vi "LPF (SubVI).vi"(9 "ZeroDimension":i32=4000, 10 "ФНЧ":bool, 11 "In":dbl[](array[numeric])) -> (3 "Filtered X":dbl[](array[numeric]))   [LabVIEW 2017]
uses:
  <vilib>/Analysis/NI_AALPro.lvlib
  <vilib>/Analysis/NI_AALBase.lvlib
panel:
  in  "Echo":bool
  in  "first":i32
  in  "Position":i32=2050
  in  "amplitude":dbl=0.002 format="%.2p"
  in  "cycles":dbl=2.0 format="%#_13g"
  in  "samples":i32=20
  in  "last":i32
  in  "index":i32
  out "Waveform Graph":dbl[][](graph)
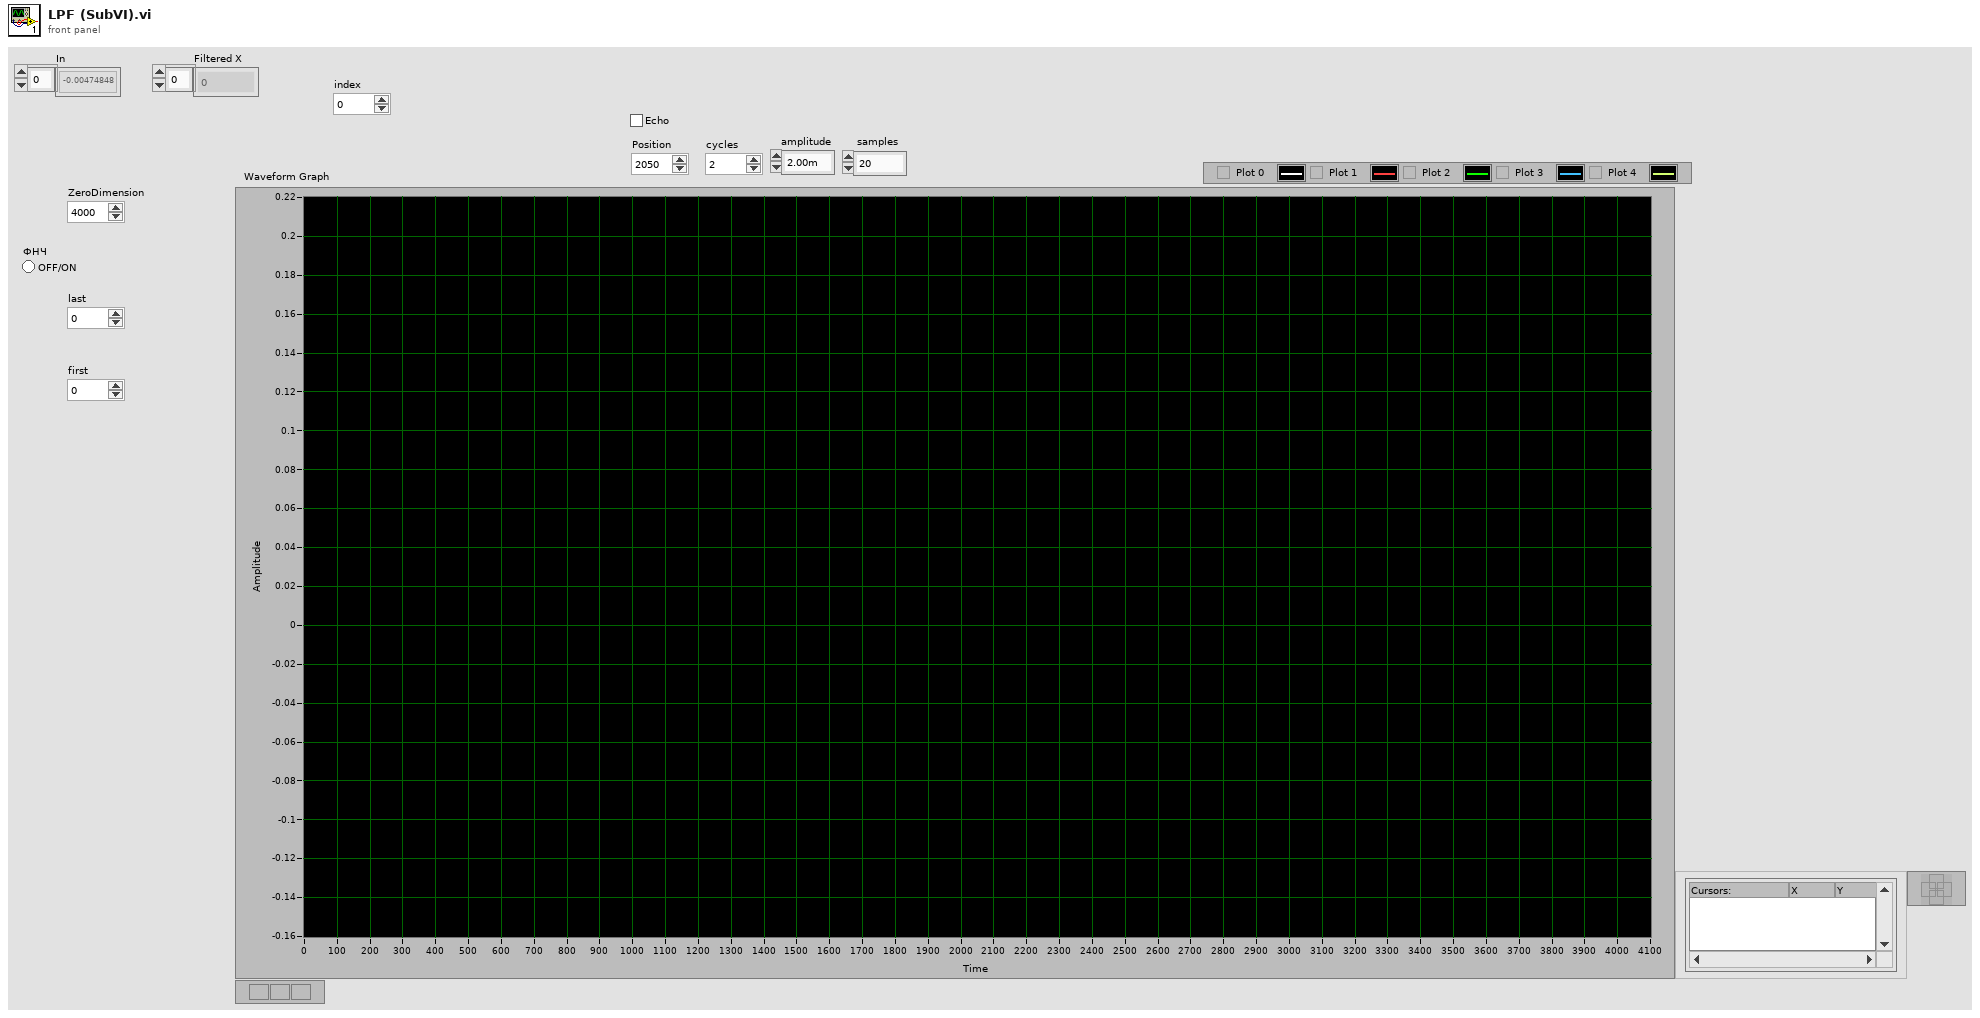
[diagram p1: front panel]
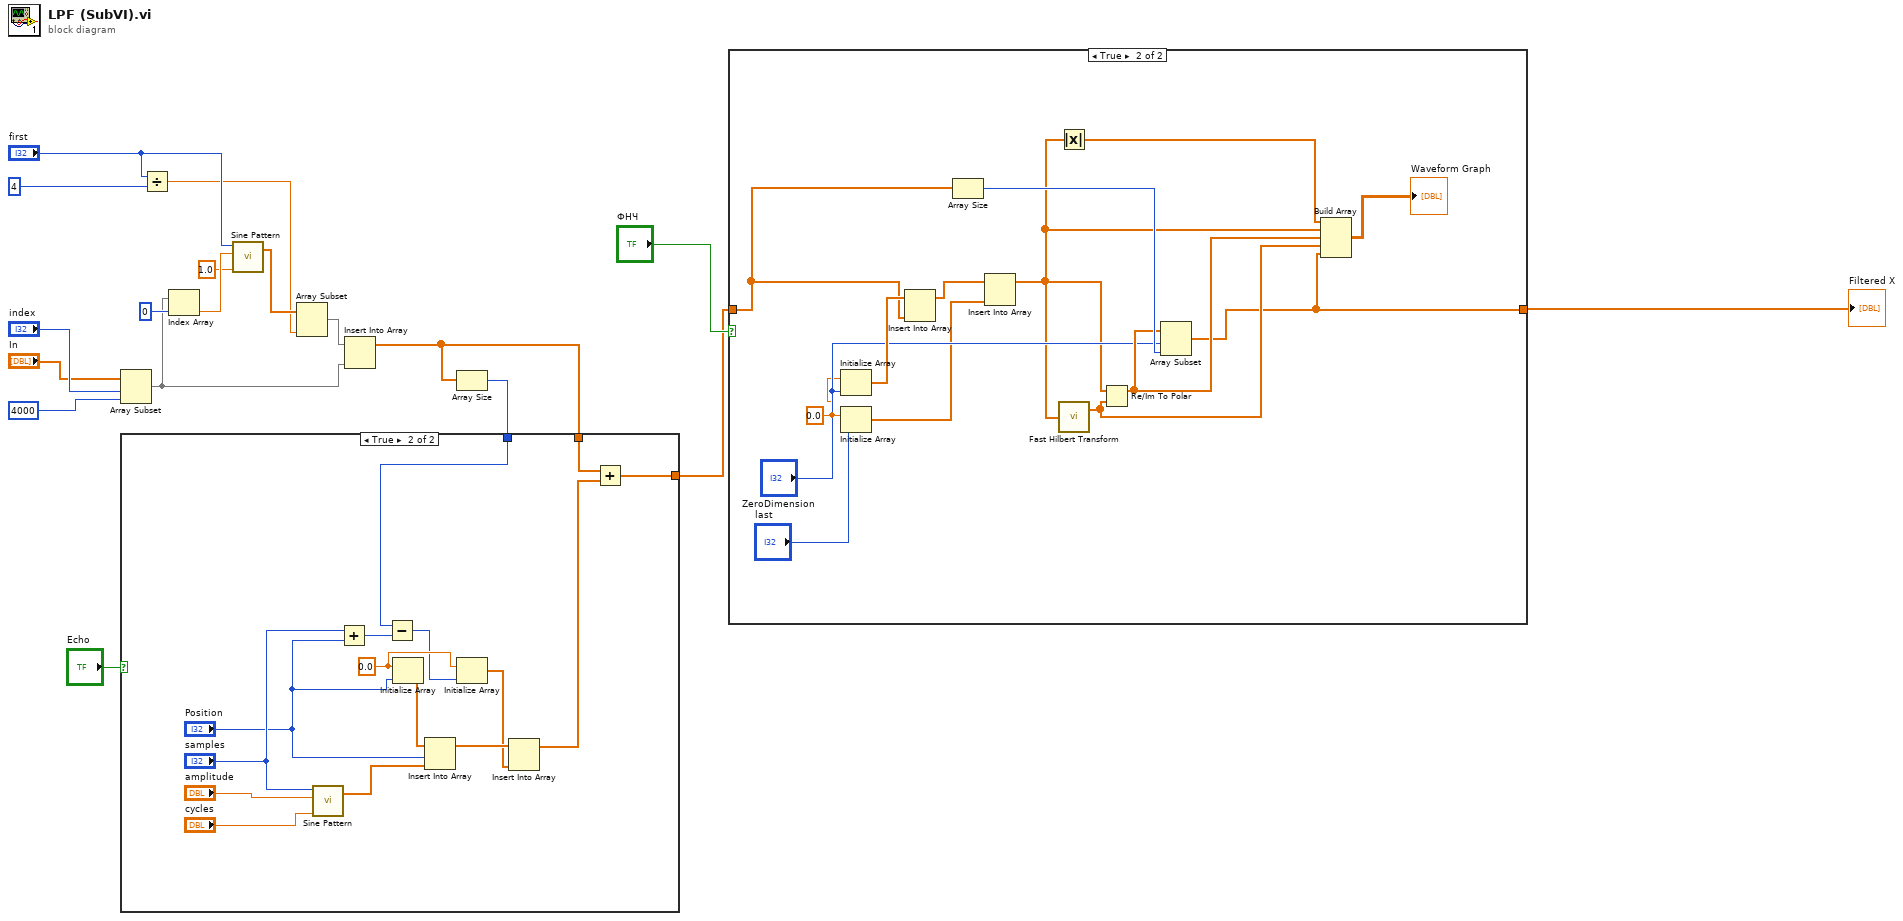
[diagram p0: block diagram]
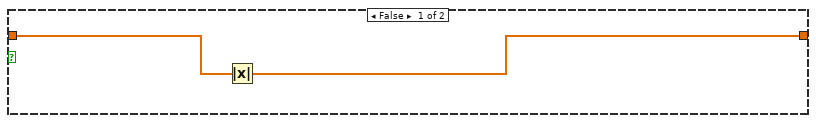
[diagram p3: hidden frame]
diagram:
  n1 = Array Subset(array="In", index="index", length=4000) -> (w3:dbl[])
  n2 = Divide(x="first", y=4) -> (x/y=w5:dbl)
  n3 = Index Array(array=w3, index=0) -> (element=w10:dbl)
  n4 = call <vilib>:"Sine Pattern.vi"("cycles"=1.0, "amplitude"=w10, "samples"="first") -> ("Sinusoidal Pattern"=w8:dbl[])  [unwired: 1 in, 1 out]
  n5 = Array Subset(array=w8, length=w5) -> (w4:dbl[])  [unwired: 1 in]
  n6 = Insert Into Array(array=w4, new element=w3) -> (w2:dbl[])  [unwired: 1 in]
  n7 = Array Size(array=w2) -> (size(s)=w13:i32)
  n8 = case shown="True" "Echo" {
    tunnel: w13 -> [_ w29]
    tunnel: [w19 w21] -> w12
    tunnel: w2 -> [w19 w20]
    frame False {
    }
    frame True {
      w30 = 0.0 ("element")
      n9 = call <vilib>:"Sine Pattern.vi"("cycles"="cycles", "amplitude"="amplitude", "samples"="samples") -> ("Sinusoidal Pattern"=w32:dbl[])  [unwired: 1 in, 1 out]
      n10 = Add(x="samples", y="Position") -> (x+y=w26:i32)
      n11 = Subtract(x=w29, y=w26) -> (x-y=w25:i32)
      n12 = Initialize Array(w30, "Position") -> (w31:dbl[])
      n13 = Insert Into Array(array=w31, index="Position", new element=w32) -> (w24:dbl[])
      n14 = Initialize Array(w30, w25) -> (w23:dbl[])
      n15 = Insert Into Array(array=w24, new element=w23) -> (w22:dbl[])  [unwired: 1 in]
      n16 = Add(x=w20, y=w22) -> (x+y=w21:dbl[])
    }
  }
  n17 = case shown="True" "ФНЧ" {
    tunnel: w12 -> [w36 w46]
    tunnel: [w35 w37] -> w17
    frame False {
      n18 = Absolute Value(x=w36) -> (abs(x)=w35:dbl[])
    }
    frame True {
      w40 = 0.0 ("element")
      n19 = Initialize Array(w40, "ZeroDimension") -> (w49:dbl[])
      n20 = Initialize Array(w40, "last") -> (w44:dbl[])
      n21 = Insert Into Array(array=w49, new element=w46) -> (w48:dbl[])  [unwired: 1 in]
      n22 = Array Size(array=w46) -> (size(s)=w50:i32)
      n23 = Insert Into Array(array=w48, new element=w44) -> (w39:dbl[])  [unwired: 1 in]
      n24 = Absolute Value(x=w39) -> (abs(x)=w38:dbl[])
      n25 = call <vilib>:"Fast Hilbert Transform.vi"("X"=w39) -> ("Hilbert{X}"=w42:dbl[])  [unwired: 1 out]
      n26 = Re/Im To Polar(2:w42, 3:w39) -> (1:w47:dbl[])  [unwired: 1 out]
      n27 = Array Subset(array=w47, index="ZeroDimension", length=w50) -> (w37:dbl[])
      n28 = Build Array(w38, w39, w47, w42, w37) -> (→"Waveform Graph":dbl[][])
    }
  }
  "Filtered X" <- w17
